vi "ALTS-2015 Robot State Controller.vi"(7 "Option":T1=enum."Enqueue State", 8 "error in":errorcluster, 11 "Enqueue State":T2=enum."Wait for Robot Availability") -> (0 "error out":errorcluster, 2 "Dequeued State":T2=enum."Wait for Robot Availability")   [LabVIEW 2013]
uses:
  Controls/ALTS-2015 Auto Program States.ctl
  ALTS-2015 Robot Cotroller Options.ctl
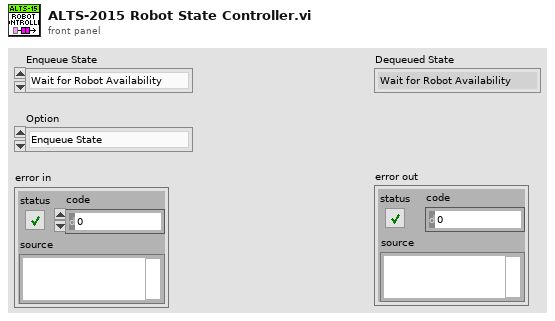
[diagram p1: front panel]
types:
  T1 = typedef "ALTS-2015 Robot Cotroller Options.ctl" = enum16{"Init", "Enqueue State", "Enqueue State in Opposite End", "Dequeue State", "Exit"}
  T2 = typedef "ALTS-2015 Auto Program States.ctl" = enum16{"<------ Robot Handler States ------>", "Wait for Robot Availability", "Wait & Read Task from Queue", "Write New Task Details to Robot", "Write Task Available for Robot", "Check Robot for Unavailbilty", "Write Task Unavailable for Robot", "<------------ Other ------------>", "Error", "Exit"}
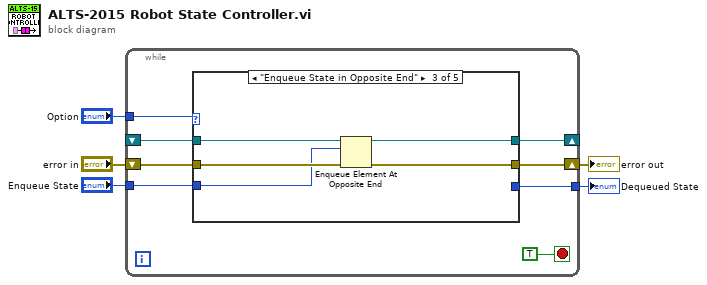
[diagram p0: block diagram]
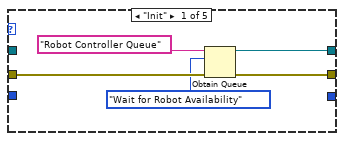
[diagram p2: hidden frame]
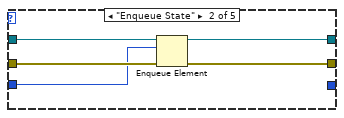
[diagram p3: hidden frame]
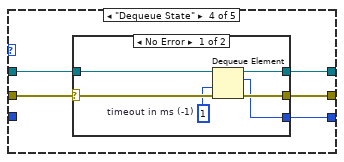
[diagram p4: hidden frame]
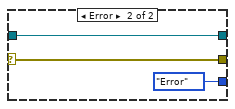
[diagram p5: hidden frame]
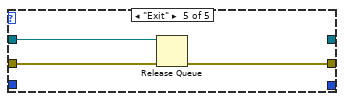
[diagram p6: hidden frame]
diagram:
  n1 = while {
    shift-right: [w13] -> _
    shift-left: _ -> [w12]
    shift-right: [w11] -> w5
    shift-left: "error in" -> [w10]
    tunnel: "Option" -> [w8]
    tunnel: "Enqueue State" -> [w7]
    tunnel: [w6] -> w2
    stop <- TRUE stop-if-true
    n2 = case shown="\"Enqueue State in Opposite End\"" w8 {
      tunnel: [w17 w20 w25 w31 _] -> w13
      tunnel: w12 -> [_ w21 w26 w32 w43]
      tunnel: [w16 w22 w27 w33 w44] -> w11
      tunnel: w10 -> [w15 w23 w28 w29 w45]
      tunnel: w7 -> [_ w19 w24 _ _]
      tunnel: [_ _ _ w30 _] -> w6
      frame "Init" {
        n3 = Obtain Queue(name (unnamed)="Robot Controller Queue", element data type=ALTS-2015_Auto_Program_States."Wait for Robot Availability", error in (no error)=w15) -> (queue out=w17:refnum<queue>, error out=w16:errorcluster)  [unwired: 2 in, 1 out]
      }
      frame "Enqueue State" {
        n4 = Enqueue Element(queue=w21, element=w19, error in (no error)=w23) -> (queue out=w20:refnum<queue>, error out=w22:errorcluster)  [unwired: 1 in, 1 out]
      }
      frame "Enqueue State in Opposite End" {
        n5 = Enqueue Element At Opposite End(queue=w26, element=w24, error in (no error)=w28) -> (queue out=w25:refnum<queue>, error out=w27:errorcluster)  [unwired: 1 in, 1 out]
      }
      frame "Dequeue State" {
        n6 = case shown="No Error" w29 {
          selector: w29 -> [w35 w41]
          tunnel: [w39 w41] -> w33
          tunnel: w32 -> [w38 w42]
          tunnel: [w37 w42] -> w31
          tunnel: [w36 ALTS-2015_Auto_Program_States."Error"] -> w30
          frame No Error {
            w34 = 1  # timeout in ms (-1)
            n7 = Dequeue Element(queue=w38, timeout in ms (-1)=w34, error in (no error)=w35) -> (queue out=w37:refnum<queue>, element=w36:T2, error out=w39:errorcluster)  [unwired: 1 out]
          }
          frame Error {
          }
        }
      }
      frame "Exit" {
        n8 = Release Queue(queue=w43, error in (no error)=w45) -> (error out=w44:errorcluster)  [unwired: 1 in, 2 out]
      }
    }
  }
  "error out" <- w5
  "Dequeued State" <- w2
